vi "initialize.vi"(8 "error in (no error)":errorcluster, 11 "PI_Piezo in":refnum<class "PI_Piezo.lvclass">) -> (0 "error out":errorcluster, 3 "PI_Piezo out":refnum<class "PI_Piezo.lvclass">)   [LabVIEW 2013, in "PI_Piezo.lvclass"]
uses:
  PI_Piezo.lvclass
  Globals.vi
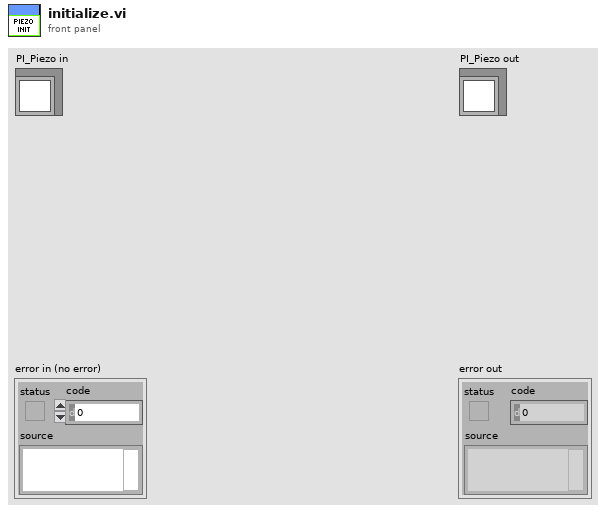
[diagram p1: front panel]
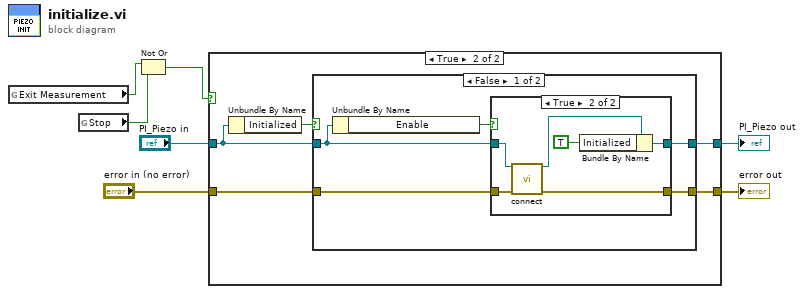
[diagram p0: block diagram]
diagram:
  n1 = global read "Globals.vi" "Exit Measurement"() -> (w3:bool)
  n2 = global read "Globals.vi" "Stop"() -> (w2:bool)
  n3 = Not Or(1:w2, 2:w3) -> (0:w1:bool)
  n4 = case shown="True" w1 {
    tunnel: [w9 w14] -> w7
    tunnel: [w8 w13] -> w6
    tunnel: "PI_Piezo in" -> [w8 w12]
    tunnel: "error in (no error)" -> [w9 w10]
    frame False {
    }
    frame True {
      n5 = Unbundle By Name(w12) -> ("Initialized"=w11:bool)
      n6 = case shown="False" w11 {
        tunnel: [w15 w28] -> w14
        tunnel: [w17 w29] -> w13
        tunnel: w12 -> [w18 w29]
        tunnel: w10 -> [w16 w28]
        frame False {
          n7 = Unbundle By Name(w18) -> ("Enable"=w19:bool)
          n8 = case shown="True" w19 {
            tunnel: w18 -> [w20 w27]
            tunnel: [w20 w23] -> w17
            tunnel: w16 -> [w21 w26]
            tunnel: [w21 w25] -> w15
            frame False {
            }
            frame True {
              n9 = call "connect.vi"("PI_Piezo.lvclass (in)"=w27, "error in"=w26) -> ("PI_Piezo.lvclass"=w24:refnum<class "PI_Piezo.lvclass">, "error out"=w25:errorcluster)  [unwired: 12 in]
              n10 = Bundle By Name(cluster=w24, "Initialized"=TRUE) -> (w23:refnum<class "PI_Piezo.lvclass">)
            }
          }
        }
        frame True {
        }
      }
    }
  }
  "error out" <- w7
  "PI_Piezo out" <- w6
